vi "End.vi"(8 "error in (no error)":errorcluster, 11 "WeatherStation in":refnum<class "WeatherStation.lvclass">) -> (0 "error out":errorcluster, 3 "WeatherStation out":refnum<class "WeatherStation.lvclass">)   [LabVIEW 2018, in "WeatherStation.lvclass"]
uses:
  WeatherStation.lvclass
  Server/Server.lvclass
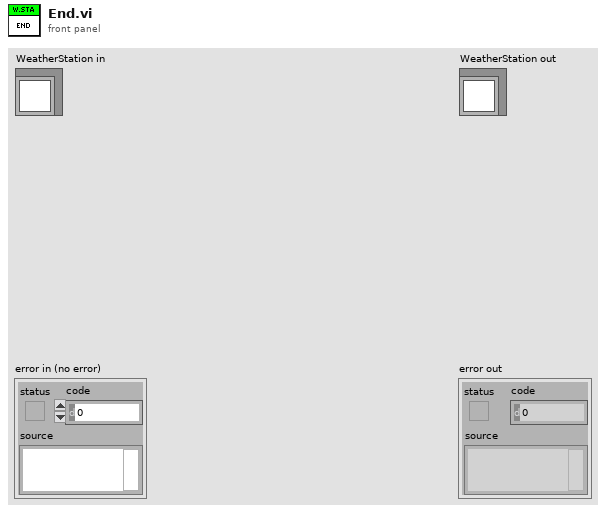
[diagram p1: front panel]
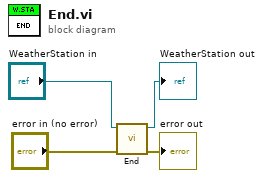
[diagram p0: block diagram]
diagram:
  n1 = call-parent "End.vi"("error in (no error)"="error in (no error)", "Server in"="WeatherStation in") -> ("error out"=→"error out":errorcluster, "Server out"=→"WeatherStation out":refnum<class "WeatherStation.lvclass">)  [unwired: 8 in]
